vi "Close.vi"(8 "error in (no error)":errorcluster, 11 "Inst.Xeryon-Rotator in":refnum<class "Inst.Xeryon-Rotator.lvclass">) -> (0 "error out":errorcluster, 3 "Inst.Xeryon-Rotator out":refnum<class "Inst.Xeryon-Rotator.lvclass">)   [LabVIEW 2019, in "Inst.Xeryon-Rotator.lvclass"]
uses:
  Inst.Xeryon-Rotator.lvclass
  C:/Program Files (x86)/National Instruments/LabVIEW 2019/user.lib/LevyLab/Instrument Framework/Instrument/Instrument.lvclass
  <userlib>/LevyLab/Instrument Framework/Instrument Types/Cryostat/Instrument.Cryostat.lvclass
  <userlib>/LevyLab/Instrument Framework/Instrument/Instrument.lvclass
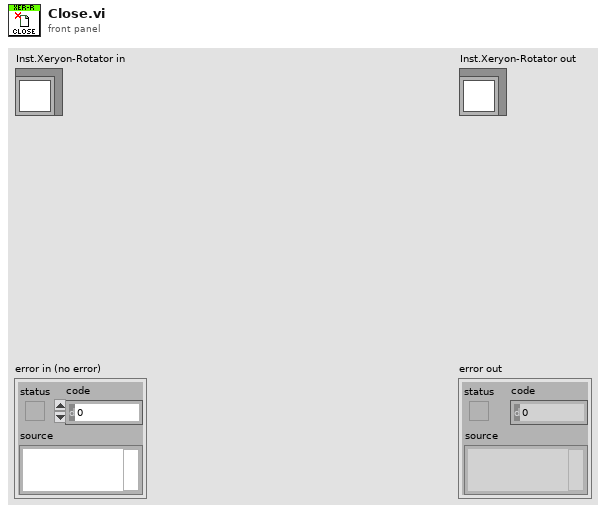
[diagram p1: front panel]
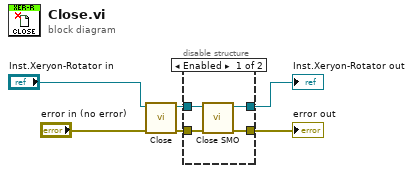
[diagram p0: block diagram]
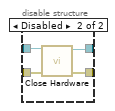
[diagram p2: hidden frame]
diagram:
  n1 = call-parent "Close.vi"("error in (no error)"="error in (no error)", "Instrument in"="Inst.Xeryon-Rotator in") -> ("error out"=w4:errorcluster, "Instrument out"=w3:refnum<class "Inst.Xeryon-Rotator.lvclass">)  [unwired: 8 in]
  n2 = disable-structure shown="Enabled" {
    disable-tunnel: w4 -> [w10 w11]
    disable-tunnel: w3 -> [w9 w14]
    disable-tunnel: [w8 w13] -> w2
    disable-tunnel: [w7 w12] -> w1
    frame Enabled {
      n3 = call <userlib>:"Close SMO.vi"("error in (no error)"=w10, "Instrument in"=w9) -> ("error out"=w7:errorcluster, "Instrument out"=w8:refnum<class "Inst.Xeryon-Rotator.lvclass">)  [unwired: 8 in]
    }
    frame Disabled {
      n4 = call-dynamic "Close Hardware.vi"("error in (no error)"=w11, "Inst.Xeryon-Rotator in"=w14) -> ("error out"=w12:errorcluster, "Inst.Xeryon-Rotator out"=w13:refnum<class "Inst.Xeryon-Rotator.lvclass">)  [unwired: 8 in]
    }
  }
  "error out" <- w1
  "Inst.Xeryon-Rotator out" <- w2
